vi "total experiment_No.vi"() -> ()   [LabVIEW 2020]
panel:
  in  "total experiment_No":i32
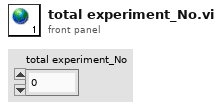
[diagram p1: front panel]
diagram:
